vi "CONST AI DAQ Settings KeyName.vi"(6 "AI TaskName":string) -> (7 "AI DAQ Settings (KeyName)":string)   [LabVIEW 2017, in "DAQ.lvclass"]
doc: "Developed by Kevin Thompson\nkevin@thompsonengineering.net\n\nCopyright 2018-2020\nThompson Engineering, LLC"
uses:
  DAQ.lvclass
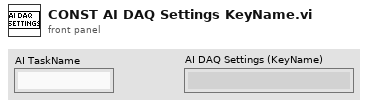
[diagram p1: front panel]
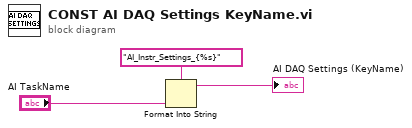
[diagram p0: block diagram]
diagram:
  n1 = Format Into String(format string="AI_Instr_Settings_{%s}" ("string"), "AI TaskName") -> (resulting string=→"AI DAQ Settings (KeyName)":string)  [unwired: 2 in, 1 out]
